vi "CreatePublicEvents.vi"(8 "error in (no error)":errorcluster, 11 "Instrument.DAQ":refnum<class "Instrument.DAQ.lvclass">) -> (0 "error out":errorcluster, 3 "Instrument.DAQ out":refnum<class "Instrument.DAQ.lvclass">)   [LabVIEW 2019, in "Instrument.Lockin.lvlib" / "Instrument.DAQ.lvclass"]
doc: "---------------------------------------------------------------\nJKI State Machine Objects™\nhttp://jki.net/state-machine-objects/\nCopyright (C) 2005-2015, JKI <info@jki.net>\nALL RIGHTS RESERVEDJKI State Machine Objects (SMO) 1.0.0.4\nJKI - JKI\nCopyright (c) 2015, JKI"
uses:
  Instrument.DAQ.lvclass
  Typedefs/PublicEvents--DAQ.getWaveforms.ctl
  Typedefs/PublicEvents--DAQ.getResults.ctl
  Typedefs/Results--Cluster.ctl
  Typedefs/PublicEvents--DAQ.getCalibration.ctl
  Typedefs/DAQ.Calibration--Cluster--Array.ctl
  Typedefs/DAQ.Calibration--Cluster.ctl
  Typedefs/PublicEvents--DAQ.getAOChannels.ctl
  Typedefs/AO.Channel--Cluster--Array.ctl
  Typedefs/AO.Channel--Cluster.ctl
  Typedefs/AO.Channel.Function--Enum.ctl
  Typedefs/PublicEvents--DAQ.getREFChannels.ctl
  Typedefs/REF.Channel--Cluster--Array.ctl
  Typedefs/REF.Channel--Cluster.ctl
  Typedefs/PublicEvents--DAQ.getDAQState.ctl
  Typedefs/Status--enum.ctl
  Typedefs/PublicEvents--DAQ.getSweepWaveforms.ctl
  Typedefs/PublicEvents--DAQ.getDAQconfig.ctl
  Typedefs/DAQ.Configuration--Cluster--Array.ctl
  Typedefs/DAQ.Configuration--Cluster.ctl
  Typedefs/DAQ.Config.AO.Range--enum.ctl
  Typedefs/DAQ.TerminalConfiguration--ring.ctl
  Typedefs/DAQ.Config.AI.Range--enum.ctl
  Typedefs/DAQ.Config.AI.Coupling--enum.ctl
  Typedefs/PublicEvents--DAQ.getAIChannels.ctl
  Typedefs/AI.Channel--Cluster--Array.ctl
  Typedefs/AI.Channel--Cluster.ctl
  Typedefs/PublicEvents--DAQ.getInputGain.ctl
  Typedefs/Channel.Gain--Cluster--Array.ctl
  Typedefs/Channel.Gain--Cluster.ctl
  Typedefs/PublicEvents--DAQ.getOutputGain.ctl
  Typedefs/PublicEvents--DAQ.getInputOffset.ctl
  Typedefs/PublicEvents--DAQ.getSampling.ctl
  Typedefs/DAQ.Sampling--Cluster.ctl
  Typedefs/DAQ.Sampling.Sampling--Cluster.ctl
  Typedefs/PublicEvents--DAQ.getSweepChannels.ctl
  Typedefs/Sweep.Configuration--Cluster.ctl
  Typedefs/Sweep.Channel--Cluster--Array.ctl
  Typedefs/Sweep.Channel--Cluster.ctl
  Typedefs/Sweep.Pattern--Enum.ctl
  Typedefs/PublicEvents--DAQ.getDeviceIDN.ctl
  Typedefs/DeviceInfo--Cluster.ctl
  Instrument.DAQ.lvclass/Instrument.DAQ.ctl
  <vilib>/JKI/JKI SMO/SMO/SMO.lvclass
panel:
  # "For instructions on how to use the JKI State Machine Objects, examples and video tutorials, visit:\nhttp://jki.net/state-machine-objects/\n\nJKI State Machine Objects™\nhttp://jki.net/state-machine-objects/\nCopyright (C) 2005-2015, JKI <info@jki.net>\nALL RIGHTS RESERVED"
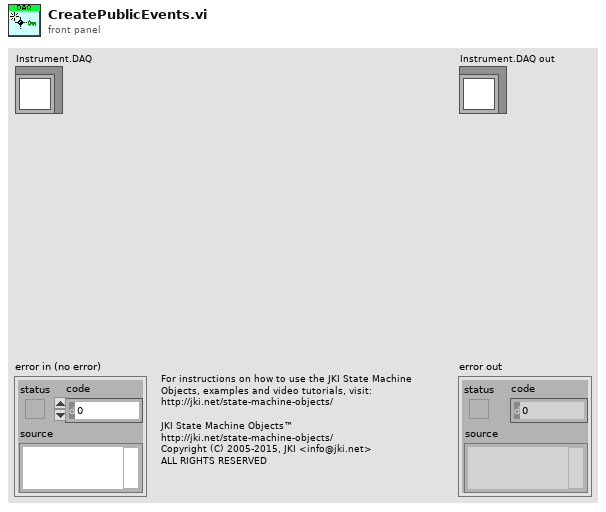
[diagram p1: front panel]
types:
  T1 = typedef "Instrument.Lockin.lvlib/Instrument.DAQ.lvclass/PublicEvents--DAQ.getDeviceIDN.ctl" = cluster{"Devices":T2[]}
  T2 = typedef "Instrument.Lockin.lvlib/Instrument.DAQ.lvclass/DeviceInfo--Cluster.ctl" = cluster{"DeviceName":string, "DevIsSimulated":bool, "DeviceSerialNumber":string, "ProductType":string, "ProductCategory":i32, "ProductNumber":u32, "ChassisNumber":u32, "SlotNumber":u32, "ChassisName":string, "ChassisSerialNumber":string, "DevTemp":dbl, "SelfCal.LastDate/Time":string, "SelfCal.LastTemp":dbl, "calibration due?":bool}
  T3 = typedef "Instrument.Lockin.lvlib/Instrument.DAQ.lvclass/PublicEvents--DAQ.getSweepChannels.ctl" = cluster{"Channels.Sweep":T4}
  T4 = typedef "Instrument.Lockin.lvlib/Instrument.DAQ.lvclass/Sweep.Configuration--Cluster.ctl" = cluster{"sweepTime":dbl, "initialWaitTime":dbl, "returnToStart":bool, "sweepChannels":T5}
  T5 = typedef "Instrument.Lockin.lvlib/Instrument.DAQ.lvclass/Sweep.Channel--Cluster--Array.ctl" = T6[]
  T6 = typedef "Instrument.Lockin.lvlib/Instrument.DAQ.lvclass/Sweep.Channel--Cluster.ctl" = cluster{"Enable?":bool, "Channel":u16, "Start":dbl, "End":dbl, "Pattern":T7, "Table":dbl[]}
  T7 = typedef "Instrument.Lockin.lvlib/Instrument.DAQ.lvclass/Sweep.Pattern--Enum.ctl" = enum16{"Ramp /", "Ramp /\\", "Smooth Ramp _/", "Smooth Ramp _/\\_", "Table"}
  T8 = typedef "Instrument.Lockin.lvlib/Instrument.DAQ.lvclass/PublicEvents--DAQ.getSampling.ctl" = cluster{"Sampling":T9}
  T9 = typedef "Instrument.Lockin.lvlib/Instrument.DAQ.lvclass/DAQ.Sampling--Cluster.ctl" = cluster{"Sampling":T10, "Fs_Out":dbl}
  T10 = typedef "Instrument.Lockin.lvlib/Instrument.DAQ.lvclass/DAQ.Sampling.Sampling--Cluster.ctl" = cluster{"Fs":dbl, "#s":i32}
  T11 = typedef "Instrument.Lockin.lvlib/Instrument.DAQ.lvclass/PublicEvents--DAQ.getInputOffset.ctl" = cluster{"Input Offset":T12}
  T12 = typedef "Instrument.Lockin.lvlib/Instrument.DAQ.lvclass/Channel.Gain--Cluster--Array.ctl" = T13[]
  T13 = typedef "Instrument.Lockin.lvlib/Instrument.DAQ.lvclass/Channel.Gain--Cluster.ctl" = cluster{"Channel":string, "Gain":dbl}
  T14 = typedef "Instrument.Lockin.lvlib/Instrument.DAQ.lvclass/PublicEvents--DAQ.getOutputGain.ctl" = cluster{"Output Gain":T12}
  T15 = typedef "Instrument.Lockin.lvlib/Instrument.DAQ.lvclass/PublicEvents--DAQ.getInputGain.ctl" = cluster{"Input Gain":T12}
  T16 = typedef "Instrument.Lockin.lvlib/Instrument.DAQ.lvclass/PublicEvents--DAQ.getAIChannels.ctl" = cluster{"Channels.AI":T17}
  T17 = typedef "Instrument.Lockin.lvlib/Instrument.DAQ.lvclass/AI.Channel--Cluster--Array.ctl" = T18[]
  T18 = typedef "Instrument.Lockin.lvlib/Instrument.DAQ.lvclass/AI.Channel--Cluster.ctl" = cluster{"Enable?":bool, "Channel":i32, "References":u16[], "reference index":i32}
  T19 = typedef "Instrument.Lockin.lvlib/Instrument.DAQ.lvclass/PublicEvents--DAQ.getDAQconfig.ctl" = cluster{"New Ch []":T20}
  T20 = typedef "Instrument.Lockin.lvlib/Instrument.DAQ.lvclass/DAQ.Configuration--Cluster--Array.ctl" = T21[]
  T21 = typedef "Instrument.Lockin.lvlib/Instrument.DAQ.lvclass/DAQ.Configuration--Cluster.ctl" = cluster{"Device":string, "Lockin.AO":string, "AO.Ch":string, "AO.Range":T22, "AO terminal config":T23, "Lockin.AI":string, "AI.Ch":string, "AI.Range":T24, "AI.Coupling":T25, "AI terminal config":T23}
  T22 = typedef "Instrument.Lockin.lvlib/Instrument.DAQ.lvclass/DAQ.Config.AO.Range--enum.ctl" = enum16{"±0.1", "±1.0", "±3.5", "±10.0", ""}
  T23 = typedef "Instrument.Lockin.lvlib/Instrument.DAQ.lvclass/DAQ.TerminalConfiguration--ring.ctl" = i32
  T24 = typedef "Instrument.Lockin.lvlib/Instrument.DAQ.lvclass/DAQ.Config.AI.Range--enum.ctl" = enum16{"±0.316", "±1.00", "±3.16", "±10.0", "±31.6", "±42.4", ""}
  T25 = typedef "Instrument.Lockin.lvlib/Instrument.DAQ.lvclass/DAQ.Config.AI.Coupling--enum.ctl" = u16
  T26 = typedef "Instrument.Lockin.lvlib/Instrument.DAQ.lvclass/PublicEvents--DAQ.getSweepWaveforms.ctl" = cluster{"AO":waveform(dbl)[], "AI":waveform(dbl)[], "X":waveform(dbl)[], "Y":waveform(dbl)[]}
  T27 = typedef "Instrument.Lockin.lvlib/Instrument.DAQ.lvclass/PublicEvents--DAQ.getDAQState.ctl" = cluster{"status":T28}
  T28 = typedef "Instrument.Lockin.lvlib/Instrument.DAQ.lvclass/Status--enum.ctl" = enum16{"idle", "created", "started", "stopped", "sweeping"}
  T29 = typedef "Instrument.Lockin.lvlib/Instrument.DAQ.lvclass/PublicEvents--DAQ.getREFChannels.ctl" = cluster{"Channels: REF":T30}
  T30 = typedef "Instrument.Lockin.lvlib/Instrument.DAQ.lvclass/REF.Channel--Cluster--Array.ctl" = T31[]
  T31 = typedef "Instrument.Lockin.lvlib/Instrument.DAQ.lvclass/REF.Channel--Cluster.ctl" = cluster{"Enable?":bool, "Channel":i32, "Frequency":dbl, "Phase":dbl, "TC":dbl, "Roll-Off":i32}
  T32 = typedef "Instrument.Lockin.lvlib/Instrument.DAQ.lvclass/PublicEvents--DAQ.getAOChannels.ctl" = cluster{"Channels: AO":T33}
  T33 = typedef "Instrument.Lockin.lvlib/Instrument.DAQ.lvclass/AO.Channel--Cluster--Array.ctl" = T34[]
  T34 = typedef "Instrument.Lockin.lvlib/Instrument.DAQ.lvclass/AO.Channel--Cluster.ctl" = cluster{"Enable?":bool, "Channel":i32, "Amplitude":dbl, "Offset":dbl, "Frequency":dbl, "Phase":dbl, "Function":T35, "Sweeping?":bool, "Limit AC":bool, "Limit DC?":bool, "Duty Cycle":bool}
  T35 = typedef "Instrument.Lockin.lvlib/Instrument.DAQ.lvclass/AO.Channel.Function--Enum.ctl" = enum16{"sine", "square", "triangle", "saw"}
  T36 = typedef "Instrument.Lockin.lvlib/Instrument.DAQ.lvclass/PublicEvents--DAQ.getCalibration.ctl" = cluster{"Calibration":T37}
  T37 = typedef "Instrument.Lockin.lvlib/Instrument.DAQ.lvclass/DAQ.Calibration--Cluster--Array.ctl" = T38[]
  T38 = typedef "Instrument.Lockin.lvlib/Instrument.DAQ.lvclass/DAQ.Calibration--Cluster.ctl" = cluster{"Active Device":string, "SelfCal.LastDate/Time":dbl, "SelfCal.LastTemp":dbl, "DevTemp":dbl, "calibration due?":bool}
  T39 = typedef "Instrument.Lockin.lvlib/Instrument.DAQ.lvclass/PublicEvents--DAQ.getResults.ctl" = cluster{"Results":T40}
  T40 = typedef "Instrument.Lockin.lvlib/Instrument.DAQ.lvclass/Results--Cluster.ctl" = cluster{"Time Stamp":timestamp, "Results (Dictionary)":cluster{"key":string, "value":dbl[]}[]}
  T41 = typedef "Instrument.Lockin.lvlib/Instrument.DAQ.lvclass/PublicEvents--DAQ.getWaveforms.ctl" = cluster{"AO":waveform(dbl)[], "AI":waveform(dbl)[], "REF_X":waveform(dbl)[], "REF_Y":waveform(dbl)[], "X":waveform(dbl)[], "Y":waveform(dbl)[]}
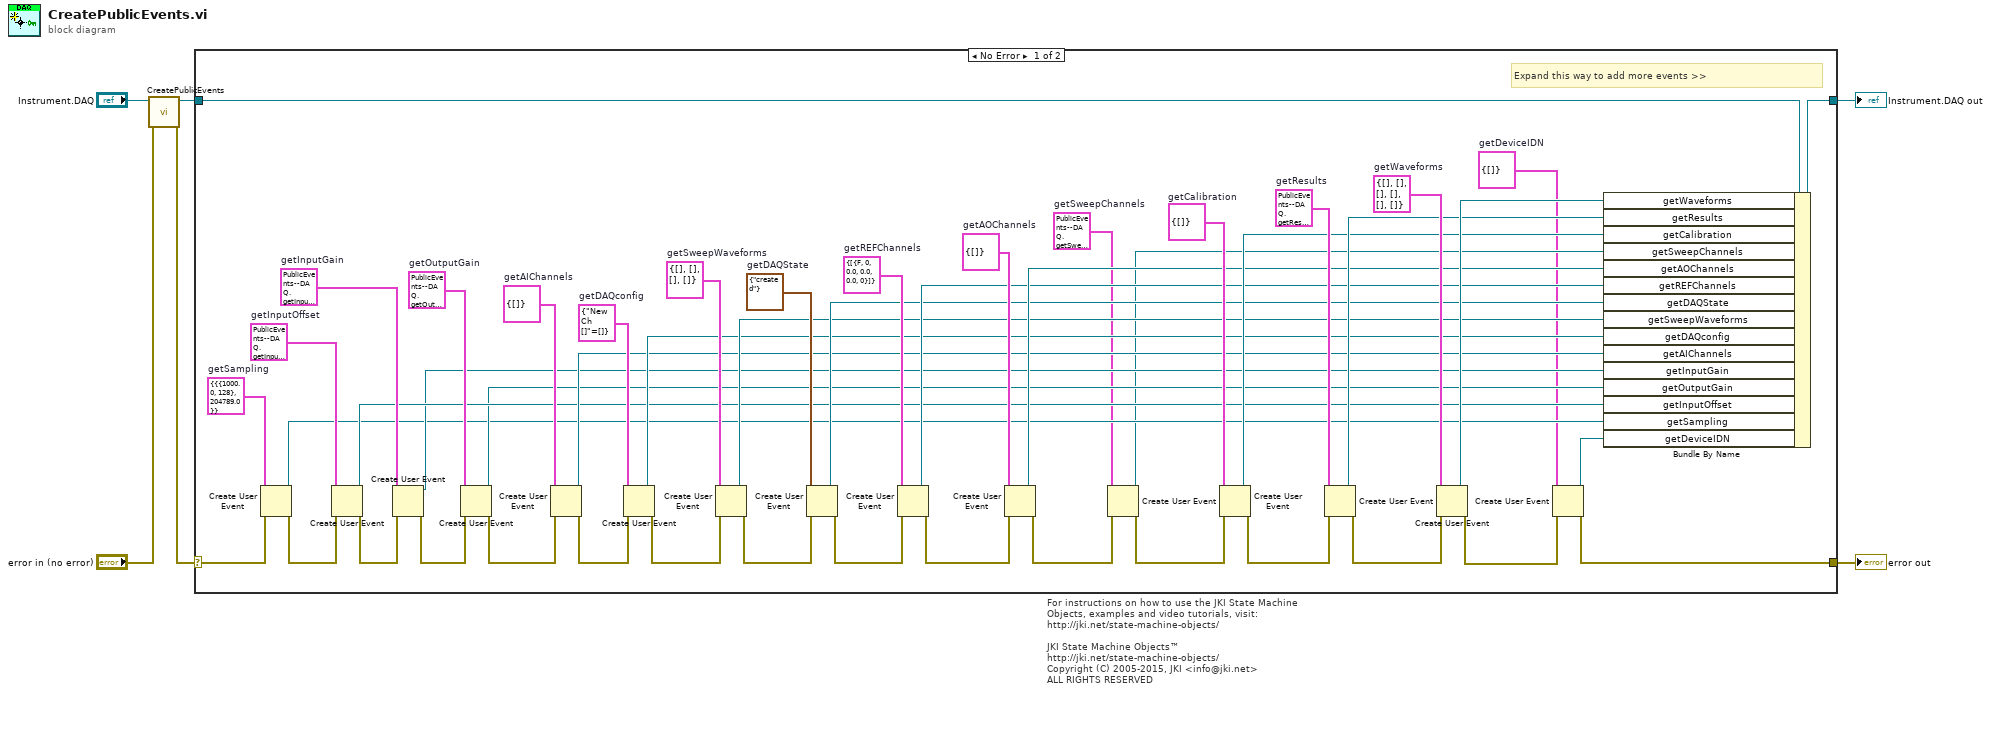
[diagram p0: block diagram]
diagram:
  # "For instructions on how to use the JKI State Machine Objects, examples and video tutorials, visit:\nhttp://jki.net/state-machine-objects/\n\nJKI State Machine Objects™\nhttp://jki.net/state-machine-objects/\nCopyright (C) 2005-2015, JKI <info@jki.net>\nALL RIGHTS RESERVED"
  n1 = call-parent "CreatePublicEvents.vi"("error in (no error)"="error in (no error)", "SMO"="Instrument.DAQ") -> ("error out"=w1:errorcluster, "SMO out"=w3:refnum<class "Instrument.DAQ.lvclass">)  [unwired: 8 in]
  n2 = case shown="No Error" w1 {
    selector: w1 -> [w17 w56]
    tunnel: [w10 w56] -> w5
    tunnel: [w53 w55] -> w6
    tunnel: w3 -> [w54 w55]
    frame No Error {
      w7 = T1 {"Devices"=[]}  # getDeviceIDN
      w14 = T3 {"Channels.Sweep"={"sweepTime"=0.0, "initialWaitTime"=0.0, "returnToStart"=FALSE, "sweepChannels"=[{"Enable?"=FALSE, "Channel"=0, "Start"=0.0, "End"=0.1, "Pattern"=enum."Ramp /", "Table"=[]}]}}  # getSweepChannels
      w18 = T8 {"Sampling"={"Sampling"={"Fs"=1000.0, "#s"=128}, "Fs_Out"=204789.0}}  # getSampling
      w23 = T11 {"Input Offset"=[{"Channel"="AI1", "Gain"=1.0}, {"Channel"="AI2", "Gain"=1.0}, {"Channel"="AI3", "Gain"=1.0}, {"Channel"="AI4", "Gain"=1.0}, {"Channel"="AI5", "Gain"=1.0}, {"Channel"="AI6", "Gain"=1.0}, {"Channel"="AI7", "Gain"=1.0}, {"Channel"="AI8", "Gain"=1.0}, {"Channel"="AI9", "Gain"=1.0}, {"Channel"="AI10", "Gain"=1.0}, {"Channel"="AI11", "Gain"=1.0}, {"Channel"="AI12", "Gain"=1.0}, {"Channel"="AI13", "Gain"=1.0}, {"Channel"="AI14", "Gain"=1.0}, {"Channel"="AI15", "Gain"=1.0}, {"Channel"="AI16", "Gain"=1.0}]}  # getInputOffset
      w24 = T14 {"Output Gain"=[{"Channel"="AI1", "Gain"=1.0}, {"Channel"="AI2", "Gain"=1.0}, {"Channel"="AI3", "Gain"=1.0}, {"Channel"="AI4", "Gain"=1.0}, {"Channel"="AI5", "Gain"=1.0}, {"Channel"="AI6", "Gain"=1.0}, {"Channel"="AI7", "Gain"=1.0}, {"Channel"="AI8", "Gain"=1.0}, {"Channel"="AI9", "Gain"=1.0}, {"Channel"="AI10", "Gain"=1.0}, {"Channel"="AI11", "Gain"=1.0}, {"Channel"="AI12", "Gain"=1.0}, {"Channel"="AI13", "Gain"=1.0}, {"Channel"="AI14", "Gain"=1.0}, {"Channel"="AI15", "Gain"=1.0}, {"Channel"="AI16", "Gain"=1.0}]}  # getOutputGain
      w25 = T15 {"Input Gain"=[{"Channel"="AI1", "Gain"=1.0}, {"Channel"="AI2", "Gain"=1.0}, {"Channel"="AI3", "Gain"=1.0}, {"Channel"="AI4", "Gain"=1.0}, {"Channel"="AI5", "Gain"=1.0}, {"Channel"="AI6", "Gain"=1.0}, {"Channel"="AI7", "Gain"=1.0}, {"Channel"="AI8", "Gain"=1.0}, {"Channel"="AI9", "Gain"=1.0}, {"Channel"="AI10", "Gain"=1.0}, {"Channel"="AI11", "Gain"=1.0}, {"Channel"="AI12", "Gain"=1.0}, {"Channel"="AI13", "Gain"=1.0}, {"Channel"="AI14", "Gain"=1.0}, {"Channel"="AI15", "Gain"=1.0}, {"Channel"="AI16", "Gain"=1.0}]}  # getInputGain
      w30 = T16 {"Channels.AI"=[]}  # getAIChannels
      w33 = T19 {"New Ch []"=[]}  # getDAQconfig
      w36 = T26 {"AO"=[], "AI"=[], "X"=[], "Y"=[]}  # getSweepWaveforms
      w38 = T27 {"status"=enum."created"}  # getDAQState
      w41 = T29 {"Channels: REF"=[{"Enable?"=FALSE, "Channel"=0, "Frequency"=0.0, "Phase"=0.0, "TC"=0.0, "Roll-Off"=0}]}  # getREFChannels
      w44 = T32 {"Channels: AO"=[]}  # getAOChannels
      w46 = T36 {"Calibration"=[]}  # getCalibration
      w49 = T39 {"Results"={"Time Stamp"=timestamp(0 s since 1904-01-01), "Results (Dictionary)"=[]}}  # getResults
      w52 = T41 {"AO"=[], "AI"=[], "REF_X"=[], "REF_Y"=[], "X"=[], "Y"=[]}  # getWaveforms
      # "Expand this way to add more events >>"
      n3 = Create User Event(user event datatype=w18, error in=w17) -> (user event=w15:refnum<user-event>, error out=w16:errorcluster)
      n4 = Create User Event(user event datatype=w23, error in=w16) -> (user event=w21:refnum<user-event>, error out=w22:errorcluster)
      n5 = Create User Event(user event datatype=w25, error in=w22) -> (user event=w19:refnum<user-event>, error out=w27:errorcluster)
      n6 = Create User Event(user event datatype=w24, error in=w27) -> (user event=w20:refnum<user-event>, error out=w26:errorcluster)
      n7 = Create User Event(user event datatype=w30, error in=w26) -> (user event=w28:refnum<user-event>, error out=w29:errorcluster)
      n8 = Create User Event(user event datatype=w33, error in=w29) -> (user event=w32:refnum<user-event>, error out=w34:errorcluster)
      n9 = Create User Event(user event datatype=w36, error in=w34) -> (user event=w35:refnum<user-event>, error out=w31:errorcluster)
      n10 = Create User Event(user event datatype=w38, error in=w31) -> (user event=w37:refnum<user-event>, error out=w39:errorcluster)
      n11 = Create User Event(user event datatype=w41, error in=w39) -> (user event=w40:refnum<user-event>, error out=w42:errorcluster)
      n12 = Create User Event(user event datatype=w44, error in=w42) -> (user event=w43:refnum<user-event>, error out=w13:errorcluster)
      n13 = Create User Event(user event datatype=w14, error in=w13) -> (user event=w11:refnum<user-event>, error out=w12:errorcluster)
      n14 = Create User Event(user event datatype=w46, error in=w12) -> (user event=w45:refnum<user-event>, error out=w47:errorcluster)
      n15 = Create User Event(user event datatype=w49, error in=w47) -> (user event=w48:refnum<user-event>, error out=w50:errorcluster)
      n16 = Create User Event(user event datatype=w52, error in=w50) -> (user event=w51:refnum<user-event>, error out=w9:errorcluster)
      n17 = Create User Event(user event datatype=w7, error in=w9) -> (user event=w8:refnum<user-event>, error out=w10:errorcluster)
      n18 = Bundle By Name(cluster=w54, "getWaveforms"=w51, "getResults"=w48, "getCalibration"=w45, "getSweepChannels"=w11, "getAOChannels"=w43, "getREFChannels"=w40, "getDAQState"=w37, "getSweepWaveforms"=w35, "getDAQconfig"=w32, "getAIChannels"=w28, "getInputGain"=w19, "getOutputGain"=w20, "getInputOffset"=w21, "getSampling"=w15, "getDeviceIDN"=w8) -> (w53:refnum<class "Instrument.DAQ.lvclass">)
    }
    frame Error {
    }
  }
  "error out" <- w5
  "Instrument.DAQ out" <- w6
